vi "Evalutation_ratio.vi"(1 "X2":dbl, 2 "X1":dbl, 3 "input cluster":cluster{"Value":dbl[], dbl[]}) -> (0 "PeaksRatio":sgl format="%#.6e")   [LabVIEW 2010]
uses:
  <vilib>/gmath/NI_Gmath.lvlib
  <vilib>/Analysis/NI_AALBase.lvlib
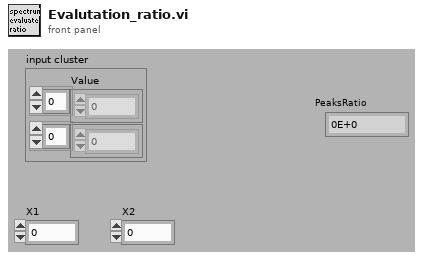
[diagram p1: front panel]
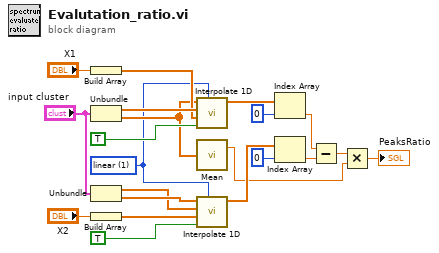
[diagram p0: block diagram]
diagram:
  w1 = 1 items=["nearest", "linear", "spline", "cubic Hermite", "Lagrange"] ("method")
  n1 = Build Array("X1") -> (w20:dbl[])
  n2 = Unbundle("input cluster") -> ("Value"=w21:dbl[], w3:dbl[])
  n3 = Unbundle("input cluster") -> ("Value"=w14:dbl[], w15:dbl[])
  n4 = Build Array("X2") -> (w13:dbl[])
  n5 = call <vilib>:"Interpolate 1D.vi"("method"=w1, "X is monotonic"=TRUE, "xi"=w20, "X"=w21, "Y"=w3) -> ("yi"=w18:dbl[])  [unwired: 4 in, 2 out]
  n6 = call <vilib>:"Mean.vi"("X"=w3) -> ("mean"=w2:dbl)  [unwired: 1 out]
  n7 = call <vilib>:"Interpolate 1D.vi"("method"=w1, "X is monotonic"=TRUE, "xi"=w13, "X"=w14, "Y"=w15) -> ("yi"=w11:dbl[])  [unwired: 4 in, 2 out]
  n8 = Index Array(array=w18, index=0) -> (element=w6:dbl)
  n9 = Index Array(array=w11, index=0) -> (element=w5:dbl)
  n10 = Subtract(x=w6, y=w5) -> (x-y=w4:dbl)
  n11 = Multiply(x=w4, y=w2) -> (x*y=→"PeaksRatio":dbl)
